vi "Camera_init.vi"(8 "error in":errorcluster, 11 "input cluster":T1={"L16 Linear Actuator"="", "XE 1000 Pump"="", "Camera1"="", "Camera2"="", "Img_Capt"=FALSE, "Actuator"=FALSE, "Pump"=FALSE, "Cam 1"=FALSE, "Cam 2"=FALSE, "Empty_Refill"=FALSE, "Crop"=FALSE, "Light intensity"=100, "Exposure Time"=1000.0, "Sample Name"="Test Sample", "Operator"="MRJ", "Calibration 1"=path "C:/Users/au540322/Desktop/IHS_Project/images/Debris/Debris_0/Debris_0_2019_06_01-23-32-49-686.PNG", "Calibration 2"=path "C:/Users/au540322/Desktop/IHS_Project/images/Debris/Debris_0/Debris_0_2019_06_01-23-32-49-686.PNG", "Framerate"=1, "Timeout Sample"=0, "Collection date"="MRJ", "Sample size threshold"=1, "Empty start"=1, "Command"="MRJ", "Station"="", "Species Name"="", "Other Notes"="", "Aperture"=enum."Item 0", "Image Process Queue Size"=500, "Image Save Queue Size"=500, "Overload threshold"=500, "Max Framerate"=100, "Rectangle 1"={"Left"=0, "Top"=0, "Right"=0, "Bottom"=0, "Rotation"=0.0}, "Rectangle 2"={"Left"=0, "Top"=0, "Right"=0, "Bottom"=0, "Rotation"=0.0}, "Detection Region %"=0.0, "Detect 1"=path "C:/Users/au540322/Desktop/IHS_Project/images/Debris/Debris_0/Debris_0_2019_06_01-23-32-49-686.PNG", "Detect 2"=path "C:/Users/au540322/Desktop/IHS_Project/images/Debris/Debris_0/Debris_0_2019_06_01-23-32-49-686.PNG", "Max large object threshold"=0, "Open(T)/Close(F)"=FALSE, "Img_Capt Begin"=FALSE, "Dispense Speed"=100, "Flush Size"=100, "Location"="Station", "Latitude"="Station", "Longitude"="Station", "Determiner"="Station", "Sex"="Station", "Camera1_Img"=refnum, "Camera2_Img"=refnum, "Img1_Orig_Disp"=refnum, "Img2_Orig_Disp"=refnum, "Img1_Orig_RGB"=refnum, "Img2_Orig_RGB"=refnum, "Blue_Plane_Extract"=refnum, "Subtracted_Plane"=refnum, "Img1_Binary"=refnum, "Img2_Binary"=refnum, "Crop_Mask"=refnum, "Img1_Save"=refnum, "Img2_Save"=refnum, "Img1_Cali_Full"=refnum, "Img2_Cali_Full"=refnum, "Img1_Cali_Detect"=refnum, "Img2_Cali_Detect"=refnum, "Cam 1 queue"=refnum, "Cam 2 queue"=refnum, "Cam 1 - save queue"=refnum, "Cam 2 - save queue"=refnum, "Overlay_Ring"=0, "SystemVersion"=0, "System Serial"=""} {"SystemVersion" items=["Standard", "XL"]; "Overlay_Ring" items=["Session Data", "Extended Setup", "Buffer", "Camera", "Dispenser", "Stats", "Connections"]; "Flush Size" min=1; "Dispense Speed" min=1; "Rectangle 2"."Rotation" format="%.2f"; "Rectangle 2"."Left" scale=0.0..1024.0; "Rectangle 2"."Right" scale=0.0..1024.0; "Rectangle 1"."Rotation" format="%.2f"; "Rectangle 1"."Left" scale=0.0..1024.0; "Rectangle 1"."Right" scale=0.0..1024.0; "Max Framerate" min=1; "Overload threshold" min=1; "Image Save Queue Size" min=1; "Image Process Queue Size" min=1; "Empty start" min=1; "Sample size threshold" min=1; "Framerate" min=1; "Light intensity" scale=0.0..100.0}) -> (0 "Cam2 Status":bool, 1 "Cam1 Status":bool, 2 "Camera2":T2, 3 "Camera1":T2)   [LabVIEW 2021]
uses:
  <vilib>/userDefined/High Color/IMAQdx.ctl
  controls/Data.ctl
  <vilib>/vision/Image Controls.llb/IMAQ Image.ctl
  <vilib>/vision/driver/IMAQdx.llb/IMAQdx Camera Control Mode.ctl
  5e997588-f8a4-47c3-81e2-b2b6234dc64e.vi
  <vilib>/vision/driver/NI_Vision_Acquisition_Software.lvlib
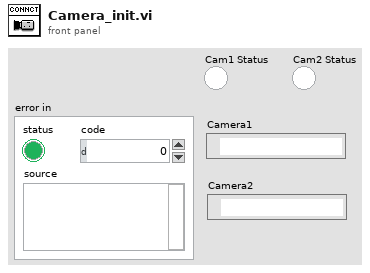
[diagram p1: front panel]
types:
  T1 = typedef "Data.ctl" = cluster{"L16 Linear Actuator":refnum<visa-resource-name>, "XE 1000 Pump":refnum<visa-resource-name>, "Camera1":T2, "Camera2":T2, "Img_Capt":bool, "Actuator":bool, "Pump":bool, "Cam 1":bool, "Cam 2":bool, "Empty_Refill":bool, "Crop":bool, "Light intensity":i32, "Exposure Time":dbl, "Sample Name":string, "Operator":string, "Calibration 1":path, "Calibration 2":path, "Framerate":i32, "Timeout Sample":i32, "Collection date":string, "Sample size threshold":i32, "Empty start":u32, "Command":string, "Station":string, "Species Name":string, "Other Notes":string, "Aperture":enum32{"Item 0", "Item 1", "Item 2", "Item 3"}, "Image Process Queue Size":i32, "Image Save Queue Size":i32, "Overload threshold":i32, "Max Framerate":i32, "Rectangle 1":T3, "Rectangle 2":T3, "Detection Region %":dbl, "Detect 1":path, "Detect 2":path, "Max large object threshold":i32, "Open(T)/Close(F)":bool, "Img_Capt Begin":bool, "Dispense Speed":i32, "Flush Size":i32, "Location":string, "Latitude":string, "Longitude":string, "Determiner":string, "Sex":string, "Camera1_Img":T4, "Camera2_Img":T4, "Img1_Orig_Disp":T4, "Img2_Orig_Disp":T4, "Img1_Orig_RGB":T4, "Img2_Orig_RGB":T4, "Blue_Plane_Extract":T4, "Subtracted_Plane":T4, "Img1_Binary":T4, "Img2_Binary":T4, "Crop_Mask":T4, "Img1_Save":T4, "Img2_Save":T4, "Img1_Cali_Full":T4, "Img2_Cali_Full":T4, "Img1_Cali_Detect":T4, "Img2_Cali_Detect":T4, "Cam 1 queue":refnum<queue>, "Cam 2 queue":refnum<queue>, "Cam 1 - save queue":refnum<queue>, "Cam 2 - save queue":refnum<queue>, "Overlay_Ring":u16, "SystemVersion":u16, "System Serial":string}
  T2 = typedef "IMAQdx.ctl" = refnum<k21>
  T3 = typedef "IMAQ Rectangle" = cluster{"Left":i32, "Top":i32, "Right":i32, "Bottom":i32, "Rotation":dbl}
  T4 = typedef "IMAQ Image.ctl" = refnum<image>
  T5 = typedef "CAM_ID.ctl" = cluster{"CAM_ID1":i32, "CAM_ID2":i32}
  T6 = typedef "NI_Vision_Acquisition_Software.lvlib/IMAQdx Camera Control Mode.ctl" = enum32{"Controller", "Listener"}
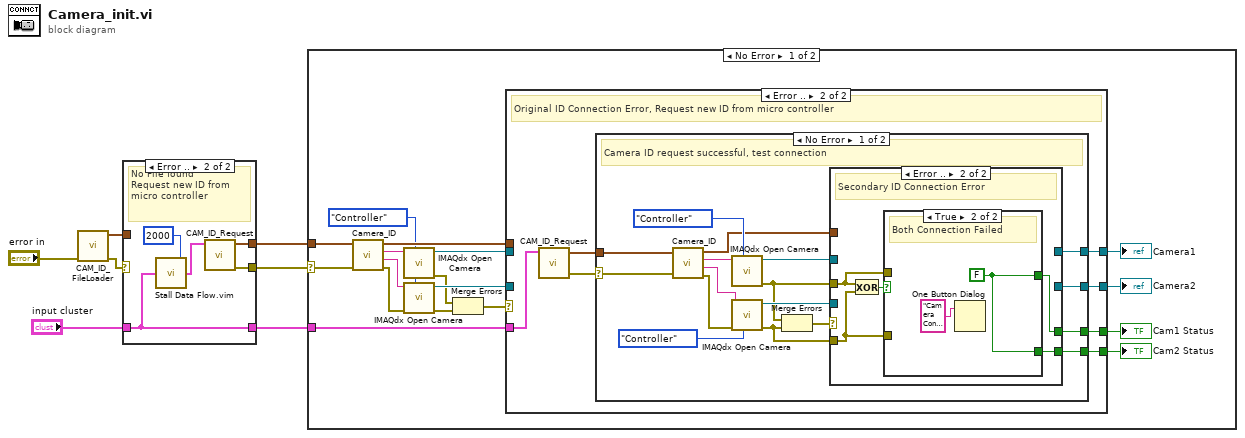
[diagram p0: block diagram]
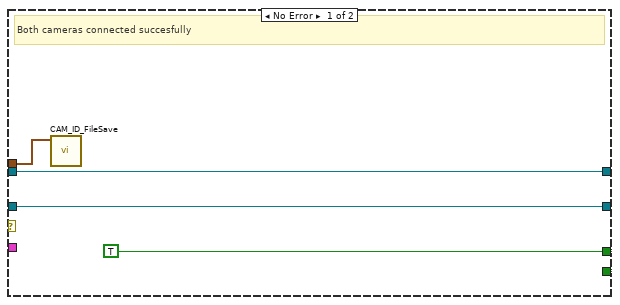
[diagram p2: hidden frame]
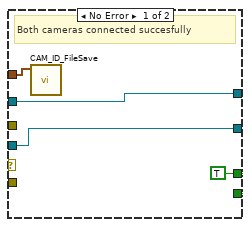
[diagram p3: hidden frame]
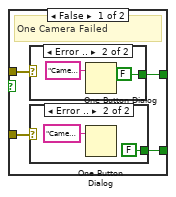
[diagram p4: hidden frame]
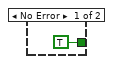
[diagram p5: hidden frame]
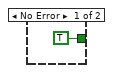
[diagram p6: hidden frame]
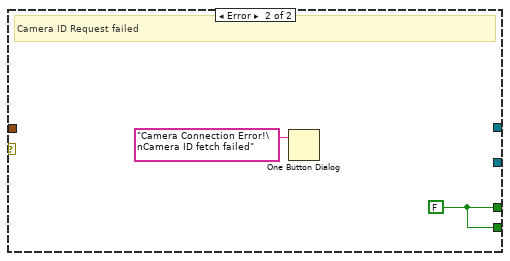
[diagram p7: hidden frame]
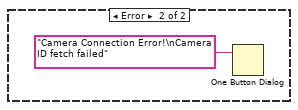
[diagram p8: hidden frame]
diagram:
  n1 = call "CAM_ID_FileLoader.vi"("error in"="error in") -> ("error out"=w5:errorcluster, "CAM_ID"=w7:T5)  [unwired: 9 in]
  n2 = case shown="Error .." w5 {
    selector: w5 -> [w9 _]
    tunnel: [w10 w15] -> w6
    tunnel: w7 -> [w10 _]
    tunnel: "input cluster" -> [w8 w11]
    tunnel: [w9 w14] -> w3
    tunnel: [w8 w11] -> w1
    frame No Error {
      # "File found"
    }
    frame Error {
      # "No File found\nRequest new ID from micro controller"
      n3 = call "Stall Data Flow.vim"("value in"=w11, "milliseconds to wait"=u32 2000) -> ("value out"=w12:T1)  [unwired: 1 out]
      n4 = call "CAM_ID_Request.vi"("input cluster"=w12) -> ("error out"=w14:errorcluster, "CAM_ID"=w15:T5)  [unwired: 9 in]
    }
  }
  n5 = case shown="No Error" w3 {
    selector: w3 -> [w28 _]
    tunnel: w6 -> [w31 _]
    tunnel: w1 -> [w21 _]
    frame No Error {
      w18 = IMAQdx_Camera_Control_Mode."Controller" ("Camera Control Mode")
      n6 = call "Camera_ID.vi"("error in"=w28, "CAM_ID"=w31) -> ("error out"=w32:errorcluster, "CAM2"=w30:string, "CAM1"=w23:string, "CAM_ID out"=w24:T5)  [unwired: 6 in]
      n7 = call <vilib>:"IMAQdx Open Camera.vi"("Camera Control Mode"=w18, "Session In"=w23) -> ("error out"=w27:errorcluster, "Session Out"=w22:T2)  [unwired: 8 in]
      n8 = call <vilib>:"IMAQdx Open Camera.vi"("Camera Control Mode"=w18, "error in"=w32, "Session In"=w30) -> ("error out"=w26:errorcluster, "Session Out"=w29:T2)  [unwired: 7 in]
      n9 = Merge Errors(w27, w26) -> (w25:errorcluster)
      n10 = case shown="Error .." w25 {
        tunnel: w29 -> [w34 _]
        tunnel: w24 -> [w36 _]
        tunnel: w22 -> [w35 _]
        tunnel: w21 -> [_ w43]
        tunnel: [w35 w41] -> w20
        tunnel: [w34 w40] -> w19
        tunnel: [w33 w39] -> w17
        tunnel: [w33 w38] -> w16
        frame No Error {
          w33 = TRUE
          # "Both cameras connected succesfully"
          n11 = call "CAM_ID_FileSave.vi"("CAM_ID"=w36) -> ()  [unwired: 11 in]
        }
        frame Error {
          # "Original ID Connection Error, Request new ID from micro controller"
          n12 = call "CAM_ID_Request.vi"("input cluster"=w43) -> ("error out"=w37:errorcluster, "CAM_ID"=w42:T5)  [unwired: 9 in]
          n13 = case shown="No Error" w37 {
            selector: w37 -> [w44 _]
            tunnel: w42 -> [w55 _]
            tunnel: [w50 _] -> w41
            tunnel: [w49 _] -> w40
            tunnel: [w46 w83] -> w39
            tunnel: [w45 w83] -> w38
            frame No Error {
              # "Camera ID request successful, test connection"
              n14 = call "Camera_ID.vi"("error in"=w44, "CAM_ID"=w55) -> ("error out"=w56:errorcluster, "CAM2"=w59:string, "CAM1"=w60:string, "CAM_ID out"=w51:T5)  [unwired: 6 in]
              n15 = call <vilib>:"IMAQdx Open Camera.vi"("Camera Control Mode"=IMAQdx_Camera_Control_Mode."Controller", "Session In"=w60) -> ("error out"=w48:errorcluster, "Session Out"=w52:T2)  [unwired: 8 in]
              n16 = call <vilib>:"IMAQdx Open Camera.vi"("Camera Control Mode"=IMAQdx_Camera_Control_Mode."Controller", "error in"=w56, "Session In"=w59) -> ("error out"=w47:errorcluster, "Session Out"=w53:T2)  [unwired: 7 in]
              n17 = Merge Errors(w48, w47) -> (w54:errorcluster)
              n18 = case shown="Error .." w54 {
                tunnel: w53 -> [w62 _]
                tunnel: w52 -> [w63 _]
                tunnel: w51 -> [w64 _]
                tunnel: [w63 _] -> w50
                tunnel: [w62 _] -> w49
                tunnel: w48 -> [_ w68]
                tunnel: w47 -> [_ w67]
                tunnel: [w61 w65] -> w46
                tunnel: [w61 w66] -> w45
                frame No Error {
                  w61 = TRUE
                  # "Both cameras connected succesfully"
                  n19 = call "CAM_ID_FileSave.vi"("CAM_ID"=w64) -> ()  [unwired: 11 in]
                }
                frame Error {
                  # "Secondary ID Connection Error"
                  n20 = Exclusive Or(1:w67, 2:w68) -> (0:w69:bool)
                  n21 = case shown="True" w69 {
                    tunnel: w68 -> [w73 _]
                    tunnel: w67 -> [w72 _]
                    tunnel: [w71 w81] -> w66
                    tunnel: [w70 w81] -> w65
                    frame False {
                      # "One Camera Failed"
                      n22 = case shown="Error .." w73 {
                        tunnel: [TRUE FALSE] -> w71
                        frame No Error {
                        }
                        frame Error {
                          n23 = One Button Dialog(message="Camera 1 connection error") -> ()  [unwired: 1 in, 1 out]
                        }
                      }
                      n24 = case shown="Error .." w72 {
                        tunnel: [TRUE FALSE] -> w70
                        frame No Error {
                        }
                        frame Error {
                          n25 = One Button Dialog(message="Camera 2 connection error") -> ()  [unwired: 1 in, 1 out]
                        }
                      }
                    }
                    frame True {
                      w81 = FALSE
                      # "Both Connection Failed"
                      n26 = One Button Dialog(message="Camera Connection Error!\nCamera Connect Failed") -> ()  [unwired: 1 in, 1 out]
                    }
                  }
                }
              }
            }
            frame Error {
              w83 = FALSE
              # "Camera ID Request failed"
              n27 = One Button Dialog(message="Camera Connection Error!\nCamera ID fetch failed") -> ()  [unwired: 1 in, 1 out]
            }
          }
        }
      }
      "Camera1" <- w20
      "Camera2" <- w19
      "Cam1 Status" <- w16
      "Cam2 Status" <- w17
    }
    frame Error {
      n28 = One Button Dialog(message="Camera Connection Error!\nCamera ID fetch failed") -> ()  [unwired: 1 in, 1 out]
    }
  }
